vi "Position Check Tester.vi"() -> ()   [LabVIEW 2018]
uses:
  Pane Position Enum.ctl
  Direction Ctl.ctl
  Boolean Object.lvclass/Boolean Object Position.lvclass
  Pane Object Position.lvclass
panel:
  out "Direction":T1
  out "Nearest Side":T2=enum."Top"
  out "Position":T2=enum."Top"
  in  "Stop":bool
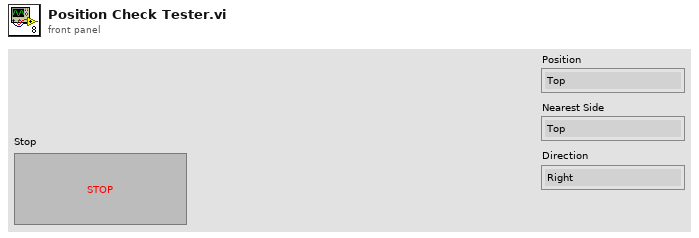
[diagram p1: front panel]
types:
  T1 = typedef "Direction Ctl.ctl" = enum16{"Right", "Left", "Up", "Down"}
  T2 = typedef "Pane Object Position.lvclass/Pane Position Enum.ctl" = enum16{"Indeterminate", "Top", "Right", "Top Right", "Bottom", "5", "Bottom Right", "7", "Left", "Top Left", "10", "11", "Bottom Left"}
  T3 = typedef "Pane Object Position.lvclass/Object Coordinates.ctl" = cluster{"Top":i32, "Right":i32, "Bottom":i32, "Left":i32}
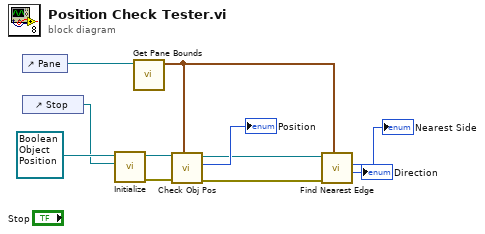
[diagram p0: block diagram]
diagram:
  n1 = control-ref of="Pane"() -> (w9:refnum<vi>)
  n2 = control-ref of="Stop"() -> (w10:refnum<vi>)
  n3 = call-dynamic "Initialize.vi"("Ctl Refnum"=w10, "Boolean Object Position in"=refnum<class "Boolean Object Position.lvclass"> refnum ("Boolean Object Position.lvclass")) -> ("error out"=w7:errorcluster, "Boolean Object Position out"=w8:refnum<class "Boolean Object Position.lvclass">)  [unwired: 8 in]
  n4 = call "Get Pane Bounds.vi"("Pane"=w9) -> ("Panel Coordinates"=w3:T3)  [unwired: 9 in, 1 out]
  n5 = call-dynamic "Check Obj Pos.vi"("Pane Coordinates"=w3, "error in (no error)"=w7, "Boolean Object Position in"=w8) -> ("error out"=w4:errorcluster, "Position"=→"Position":T2, "Boolean Object Position out"=w5:refnum<class "Boolean Object Position.lvclass">)  [unwired: 6 in]
  n6 = call-dynamic "Find Nearest Edge.vi"("Pane Coordinates"=w3, "error in (no error)"=w4, "Boolean Object Position in"=w5) -> ("Direction"=→"Direction":T1, "Nearest Side"=→"Nearest Side":T2)  [unwired: 5 in, 2 out]
